vi "SRS SR124 Lockin.vi"(1 "Action":T5=enum."Identify", 2 "Parameters":variant) -> (6 "Output":variant, 7 "Stop":bool)   [LabVIEW 2025]
doc: "Author: Scott Hannahs <sth@magnet.fsu.edu>\n\nThis software is licensed for use under the “MIT License\"\nCopyright (c) 2025 Scott Hannahs, sth@sth@magnet.sthnet.net\n\nPermission is hereby granted, free of charge, to any person obtaining a copy of this software and associated documentation files (the \"Software\"), to deal in the Software without restriction, including without limitation the rights to use, copy, modify, merge, publish, distribute, sublicense, and/or sell copies of the Software, and to permit persons to whom the Software is furnished to do so, subject to the following conditions: The above copyright notice and this permission notice shall be included in all copies or substantial portions of the Software.\n\nTHE SOFTWARE IS PROVIDED \"AS IS\", WITHOUT WARRANTY OF ANY KIND, EXPRESS OR IMPLIED, INCLUDING BUT NOT LIMITED TO THE WARRANTIES OF MERCHANTABILITY, FITNESS FOR A PARTICULAR PURPOSE AND NONINFRINGEMENT. IN NO EVENT SHALL THE AUTHORS OR COPYRIGHT HOLDERS BE LIABLE FOR ANY CLAIM, DAMAGES OR OTHER LIABILITY, WHETHER IN AN ACTION OF CONTRACT, TORT OR OTHERWISE, ARISING FROM, OUT OF OR IN CONNECTION WITH THE SOFTWARE OR THE USE OR OTHER DEALINGS IN THE SOFTWARE."
uses:
  Sub Controls/Instrument Actions.ctl
  Sub Controls/Public.ctl
  Sub Controls/Instrument Match.ctl
  SubVIs/Lockin Channels.ctl
  Sub Controls/Factory Reset.ctl
  Sub Controls/Scan Output.ctl
  Sub Controls/Instrument IDN.ctl
  Sub Controls/User Event Command.ctl
panel:
  in  "Factory Reset":T1
  out "Channel Index":i32
  in  "Channels":T2={"X"=TRUE, "X&Y"=FALSE, "R"=FALSE, "R & ϴ"=FALSE}
  out "Model 2":string
  in  "Optical Port":enum32{"Port 1", "Port 2", "Port 3", "Port 4"}(radio)
  out "Title":string="Stanford Research Analog Lockin"
  in  "VISA resource name":refnum<visa-resource-name>
  in  "Instruments":T3[](array[typedef])=[{"Model"="SR124", "Manufacturer"="Stanford_Research_Systems", "Term Character"="", "Wait Time (mS)"=0, "Wait for SRQ"=FALSE, "Type"="Lockin"}, {"Model"="SR2124", "Manufacturer"="Stanford_Research_Systems", "Term Character"="", "Wait Time (mS)"=0, "Wait for SRQ"=FALSE, "Type"="Lockin"}]
  out "Model":string
  in  "Address":u16(ring)
  in  "Public":T4
  out "Measurement":dbl[](array[numeric]) format="%^.3e"
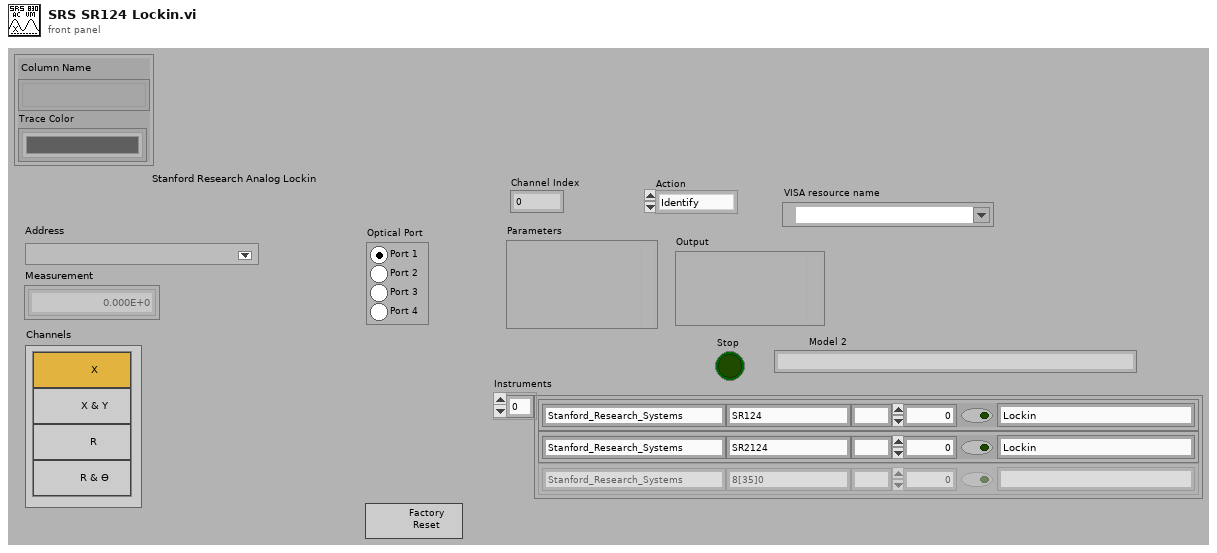
[diagram p1: front panel]
types:
  T1 = typedef "Factory Reset.ctl" = bool
  T2 = typedef "Lockin Channels.ctl" = cluster{"X":bool, "X&Y":bool, "R":bool, "R & ϴ":bool}
  T3 = typedef "Instrument Match.ctl" = cluster{"Model":string, "Manufacturer":string, "Term Character":string, "Wait Time (mS)":u32, "Wait for SRQ":bool, "Type":string}
  T4 = typedef "Public.ctl" = cluster{"Column Name":string[], "Trace Color":u32[]}
  T5 = typedef "Instrument Actions.ctl" = enum16{"Scan", "Identify", "New", "Configure", "Initialize", "Test", "Read", "Close"}
  T6 = typedef "Scan Output.ctl" = cluster{"Manufacturer":string, "Model":string, "Info":string, "Revision":string, "error out":errorcluster}
  T7 = typedef "Instrument IDN.ctl" = cluster{"VISA Address":string, "Status":u16, "Manufacturer":string, "Model":string, "Info":string, "Info 2":string, "Misc Data":variant}
  T8 = typedef "User Event Command.ctl" = enum32{"Stop Config"}
  T9 = typedef "Instrument Properties.ctl" = cluster{"Public":T4, "Private":T10}
  T10 = typedef "Private.ctl" = cluster{"Path":path, "VI Refnum":T11, "Name":string, "# of Values":i32, "Scale Factors":dbl[], "Display":T12[], "Offset":dbl[]}
  T11 = typedef "Instrument Ref.ctl" = refnum<vi>
  T12 = typedef "SystemCheckBox-resize.ctl" = bool
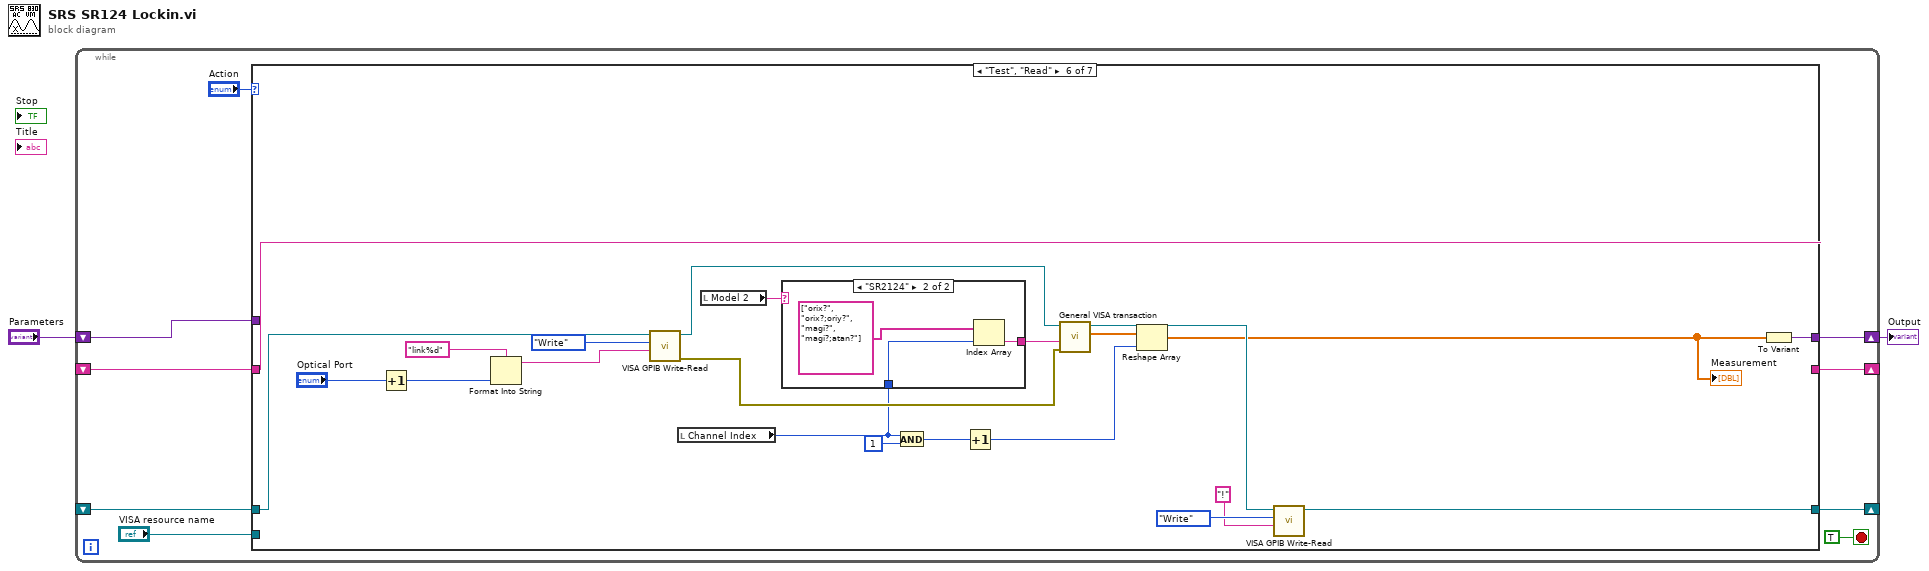
[diagram p0: block diagram]
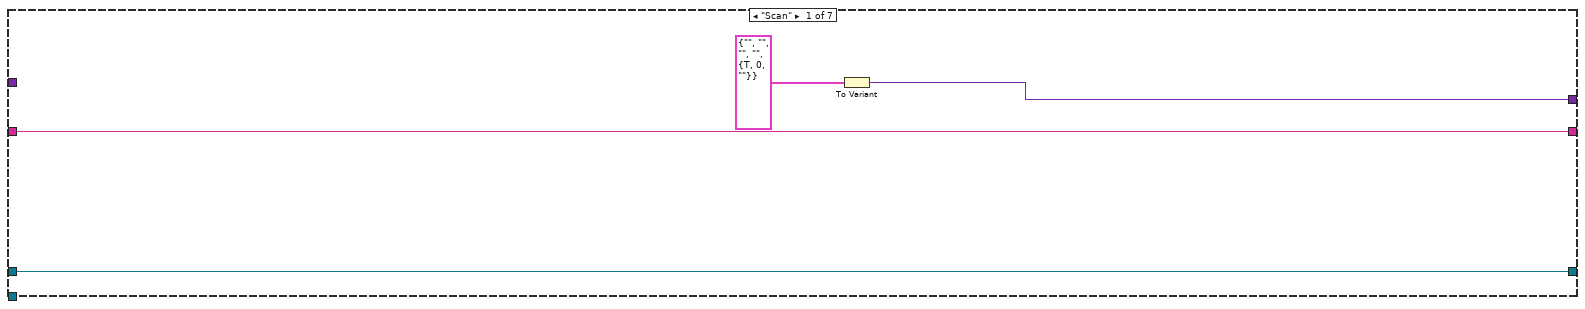
[diagram p2: hidden frame]
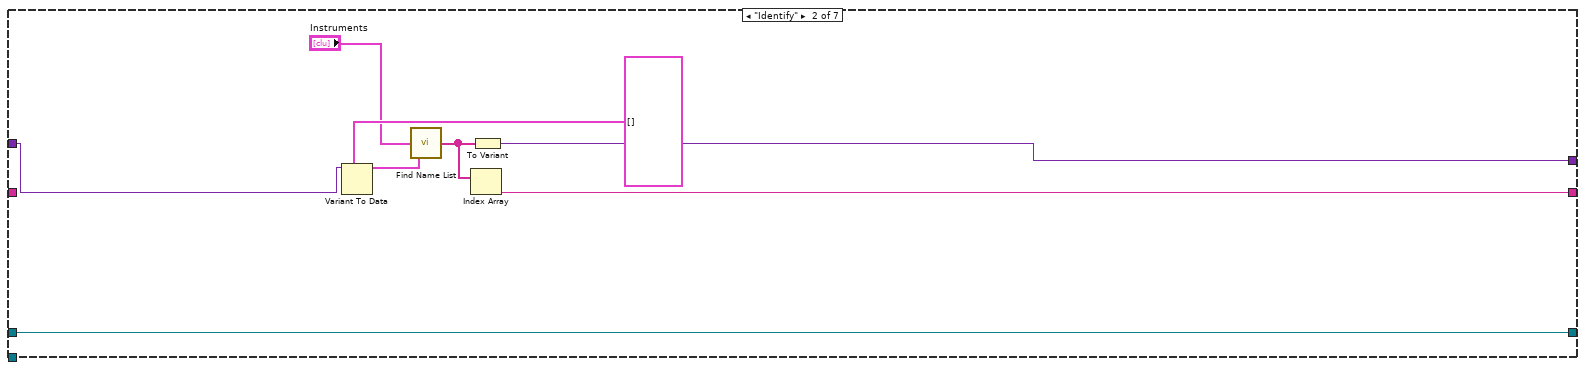
[diagram p3: hidden frame]
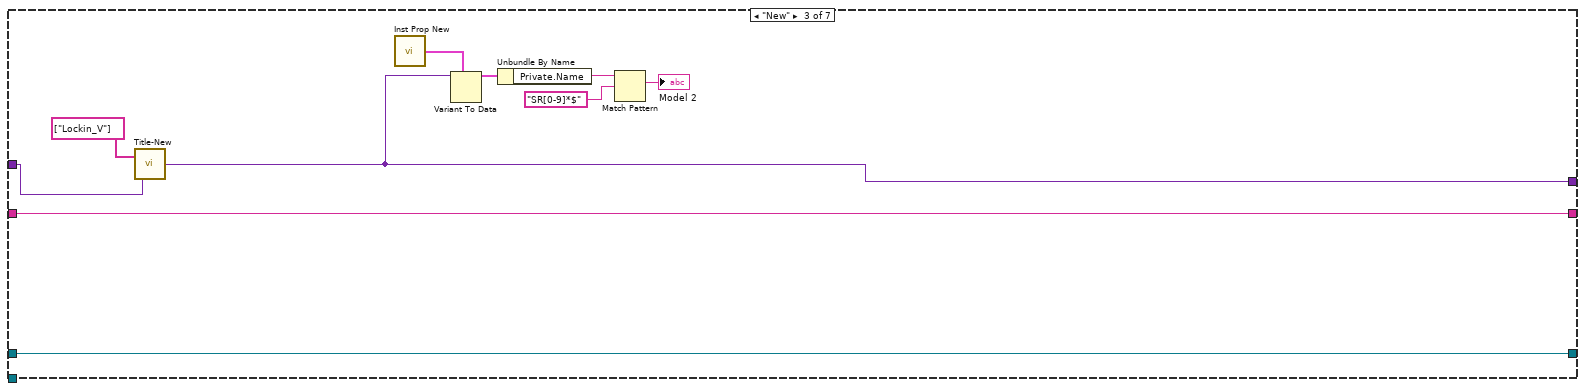
[diagram p4: hidden frame]
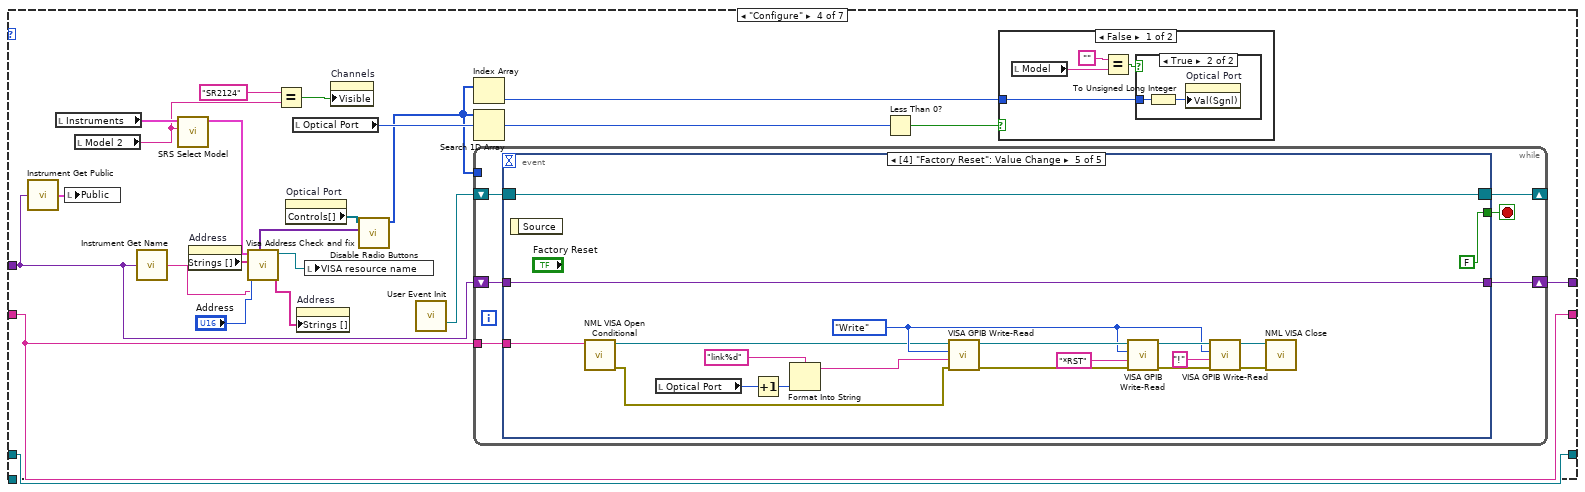
[diagram p5: hidden frame]
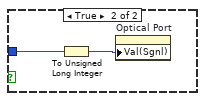
[diagram p7: hidden frame]
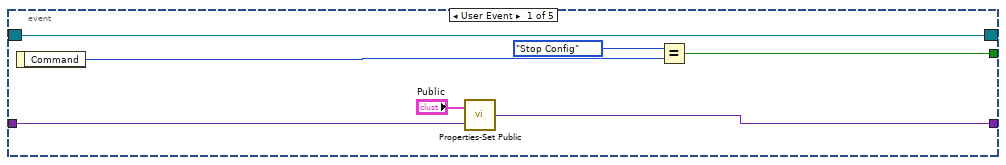
[diagram p8: hidden frame]
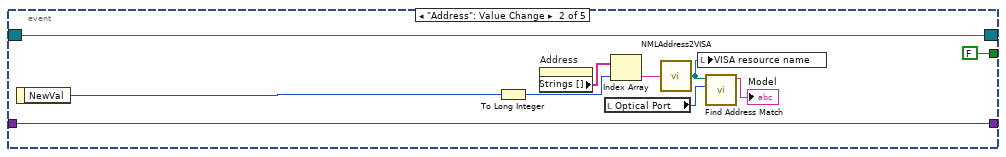
[diagram p9: hidden frame]
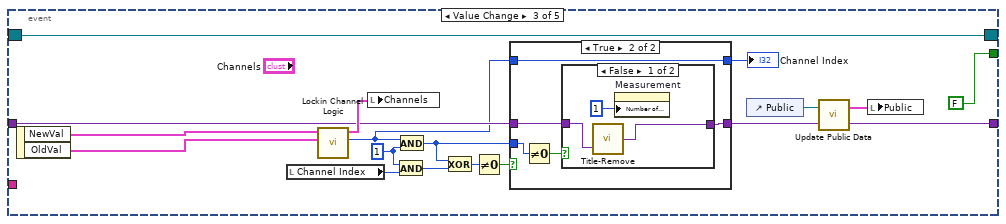
[diagram p10: hidden frame]
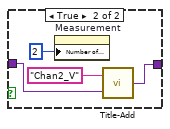
[diagram p12: hidden frame]
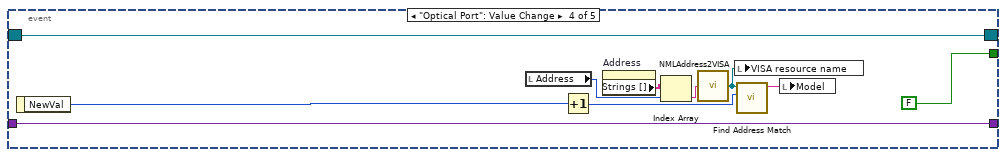
[diagram p13: hidden frame]
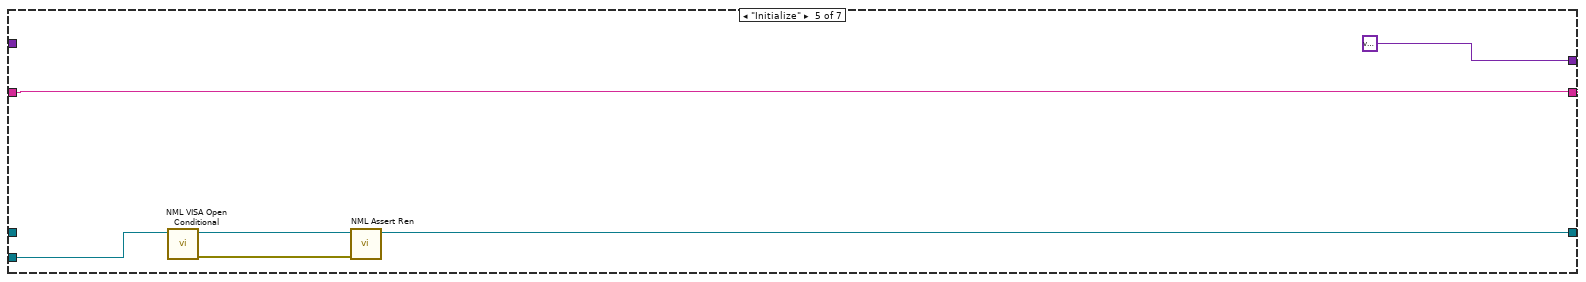
[diagram p14: hidden frame]
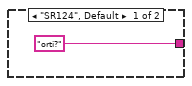
[diagram p15: hidden frame]
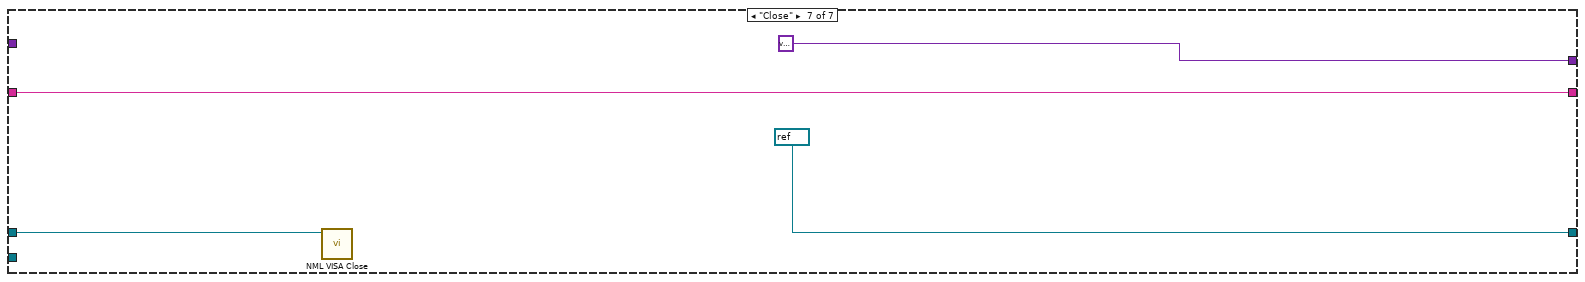
[diagram p16: hidden frame]
diagram:
  n1 = while {
    shift-right: [w10] -> _
    shift-left: _ -> [w9]
    shift-right: [w7] -> w1
    shift-left: "Parameters" -> [w8]
    shift-right: [w4] -> _
    shift-left: _ -> [w3]
    stop <- TRUE stop-if-true
    n2 = case shown="\"Test\", \"Read\"" "Action" {
      tunnel: [w14 w23 w32 w56 w150 w169 refnum<visa-resource-name> refnum ("Open VISA Resource name")] -> w10
      tunnel: w9 -> [w14 w23 w32 w56 _ w174 w181]
      tunnel: w8 -> [_ w20 w33 w47 _ _ _]
      tunnel: [w13 w22 w28 w55 variant ("Variant") w176 variant ("Variant")] -> w7
      tunnel: "VISA resource name" -> [_ _ _ _ w149 _ _]
      tunnel: [w12 w16 w30 w34 w153 w175 w182] -> w4
      tunnel: w3 -> [w12 _ w30 w34 w153 w175 w182]
      frame "Scan" {
        n3 = To Variant(anything=T6 {"Manufacturer"="", "Model"="", "Info"="", "Revision"="", "error out"={"status"=TRUE, "code"=0, "source"=""}} ("Scan Output")) -> (Variant=w13:variant)
      }
      frame "Identify" {
        n4 = Variant To Data(type=T7[] [], Variant=w20) -> (data=w18:T7[])  [unwired: 1 in, 1 out]
        n5 = call "Find Name List.vi"("Bus Scan"=w18, "Instruments"="Instruments") -> ("Names"=w17:string[])  [unwired: 1 in]
        n6 = Index Array(array=w17) -> (element=w16:string)  [unwired: 1 in]
        n7 = To Variant(anything=w17) -> (Variant=w22:variant)
      }
      frame "New" {
        n8 = call "Title-New.vi"("Parameters"=w33, "Array"=string[] ["Lockin_V"]) -> ("Instrument Prop"=w28:variant)
        n9 = call "Inst Prop New.vi"() -> ("Instrument Prop Out"=w29:T9)
        n10 = Variant To Data(type=w29, Variant=w28) -> (data=w27:T9)  [unwired: 1 in, 1 out]
        n11 = Unbundle By Name(w27) -> ("Private.Name"=w26:string)
        n12 = Match Pattern(string=w26, regular expression="SR[0-9]*$") -> (match substring=→"Model 2":string)  [unwired: 1 in, 3 out]
      }
      frame "Configure" {
        n13 = call "Instrument Get Public.vi"("Variant"=w47) -> ("Public"=w54:T4)
        n14 = local read "Instruments"() -> (w39:T3[])
        n15 = local write "Public"(w54) -> ()
        n16 = local read "Model 2"() -> (w35:string)
        n17 = call "Instrument Get Name.vi"("Parameters"=w47) -> ("Type"=w48:string)
        n18 = call "SRS Select Model.vi"("Model"=w35, "Instruments in"=w39) -> ("Instruments out"=w38:T3[])  [unwired: 9 in]
        n19 = property on="Address" class="Ring (strict)"() -> ("Strings []"=w51:string[])  [unwired: 2 in, 2 out]
        n20 = call "Visa Address Check and fix.vi"("Instruments"=w38, "NML Addresses"=w51, "Name"=w48, "Address"="Address") -> ("Array"=w46:variant[], "VISA resource name"=w50:refnum<visa-resource-name>, "NML Addresses"=w49:string[])  [unwired: 4 out]
        n21 = Equal?(x="SR2124", y=w35) -> (x = y?=w37:bool)
        n22 = property on="Optical Port" class="RadioBtnsControl (strict)"() -> ("Controls[]"=w45:refnum<vi>[])  [unwired: 2 in, 2 out]
        n23 = local read "Optical Port"() -> (w42:enum32{"Port 1", "Port 2", "Port 3", "Port 4"})
        n24 = property on="Address" class="Ring (strict)"("Strings []"=w49) -> ()  [unwired: 2 in, 2 out]
        n25 = local write "VISA resource name"(w50) -> ()
        n26 = property on="Channels" class="Clust (strict)"("Visible"=w37) -> ()  [unwired: 2 in, 2 out]
        n27 = call "Disable Radio Buttons.vi"("Array in"=w46, "Controls[]"=w45) -> ("Array out"=w41:i32[])  [unwired: 9 in]
        n28 = call "User Event Init.vi"() -> ("Event Registration Refnum"=w53:refnum<event-registration>)  [unwired: 14 in, 1 out]
        n29 = Index Array(array=w41) -> (element=w40:i32)  [unwired: 1 in]
        n30 = Search 1D Array(1D array=w41, element=w42) -> (index of element=w44:i32)  [unwired: 1 in]
        n31 = while {
          shift-right: [w70] -> w55
          shift-left: w47 -> [w69]
          shift-right: [w66] -> _
          shift-left: w53 -> [w67]
          tunnel: w41 -> [_]
          tunnel: w34 -> [w65]
          stop <- w68 stop-if-true
          n32 = event shown="[4] \"Factory Reset\": Value Change" {
            selector: w67 -> [w71 w87 w101 w129 w148]
            dyn-events: [w71 w87 w101 w129 w148] -> w66
            timeout: _ -> [_ _ _ _ _]
            tunnel: [w73 FALSE FALSE FALSE FALSE] -> w68
            tunnel: w69 -> [w76 w81 w93 w125 w147]
            tunnel: [w77 w81 w104 w125 w147] -> w70
            tunnel: w65 -> [_ _ _ _ w132]
            event User Event {
              n33 = event-data() -> ("Command"=w75:T8)  [unwired: 1 in]
              n34 = call "Properties-Set Public.vi"("Variant"=w76, "New Public"="Public") -> ("Variant 2"=w77:variant)
              n35 = Equal?(x=User_Event_Command."Stop Config", y=w75) -> (x = y?=w73:bool)
            }
            event "Address": Value Change {
              n36 = event-data() -> ("NewVal"=w85:u16)  [unwired: 1 in]
              n37 = To Long Integer(number=w85) -> (32bit integer=w79:i32)
              n38 = property on="Address" class="Ring (strict)"() -> ("Strings []"=w84:string[])  [unwired: 2 in, 2 out]
              n39 = local read "Optical Port"() -> (w78:enum32{"Port 1", "Port 2", "Port 3", "Port 4"})
              n40 = Index Array(array=w84, index=w79) -> (element=w83:string)
              n41 = call "NMLAddress2VISA.vi"("NML Address"=w83) -> ("VISA resource name"=w80:refnum<visa-resource-name>)
              n42 = local write "VISA resource name"(w80) -> ()
              n43 = call "Find Address Match.vi"("Misc Info"=w78, "VISA resource name"=w80) -> ("Model"=→"Model":string)  [unwired: 2 in, 3 out]
            }
            event Value Change {
              w98 = 1 ("y")
              n44 = event-data() -> ("NewVal"=w95:T2, "OldVal"=w94:T2)  [unwired: 1 in]
              n45 = local read "Channel Index"() -> (w99:i32)
              n46 = call "Lockin Channel Logic.vi"("Old Channels"=w94, "New Channels"=w95) -> ("index of element"=w90:i32, "Channels Out"=w100:T2)  [unwired: 8 in]
              n47 = local write "Channels"(w100) -> ()
              n48 = And(x=w98, y=w99) -> (x .and. y?=w97:i32)
              n49 = And(x=w90, y=w98) -> (x .and. y?=w91:i32)
              n50 = Exclusive Or(1:w97, 2:w91) -> (0:w96:i32)
              n51 = Not Equal To 0?(x=w96) -> (x != 0?=w92:bool)
              n52 = case shown="True" w92 {
                tunnel: w93 -> [w106 w112]
                tunnel: [w106 w111] -> w89
                tunnel: w91 -> [_ w109]
                tunnel: [w107 w108] -> w88
                tunnel: w90 -> [w107 w108]
                frame False {
                }
                frame True {
                  n53 = Not Equal To 0?(x=w109) -> (x != 0?=w110:bool)
                  n54 = case shown="False" w110 {
                    tunnel: w112 -> [w115 w119]
                    tunnel: [w114 w118] -> w111
                    frame False {
                      n55 = call "Title-Remove.vi"("Parameters"=w115) -> ("Variant"=w114:variant)  [unwired: 1 in]
                      n56 = property on="Measurement" class="Arr (strict)"("Number of Columns"=u32 1) -> ()  [unwired: 2 in, 2 out]
                    }
                    frame True {
                      n57 = property on="Measurement" class="Arr (strict)"("Number of Columns"=u32 2) -> ()  [unwired: 2 in, 2 out]
                      n58 = call "Title-Add.vi"("Parameters"=w119, "String"="Chan2_V") -> ("Variant"=w118:variant)
                    }
                  }
                }
              }
              "Channel Index" <- w88
              n59 = control-ref of="Public"() -> (w103:refnum<vi>)
              n60 = call "Update Public Data.vi"("Variant In"=w89, "Public 2"=w103) -> ("Variant Out"=w104:variant, "Public"=w102:T4)
              n61 = local write "Public"(w102) -> ()
            }
            event "Optical Port": Value Change {
              n62 = event-data() -> ("NewVal"=w122:enum32{"Port 1", "Port 2", "Port 3", "Port 4"})  [unwired: 1 in]
              n63 = local read "Address"() -> (w123:u16)
              n64 = Increment(x=w122) -> (x+1=w121:enum32{"Port 1", "Port 2", "Port 3", "Port 4"})
              n65 = property on="Address" class="Ring (strict)"() -> ("Strings []"=w127:string[])  [unwired: 2 in, 2 out]
              n66 = Index Array(array=w127, index=w123) -> (element=w126:string)
              n67 = call "NMLAddress2VISA.vi"("NML Address"=w126) -> ("VISA resource name"=w124:refnum<visa-resource-name>)
              n68 = local write "VISA resource name"(w124) -> ()
              n69 = call "Find Address Match.vi"("Misc Info"=w121, "VISA resource name"=w124) -> ("Model"=w120:string)  [unwired: 2 in, 3 out]
              n70 = local write "Model"(w120) -> ()
            }
            event Value Change {
              w136 = enum16{"Write", "Read", "Write & Read"}."Write" ("Action")
              n71 = event-data() -> ()  [unwired: 1 in, 1 out]
              n72 = call "NML VISA Open Conditional.vi"("VISA resource name"=w132) -> ("error out"=w130:errorcluster, "dup VISA Session"=w131:refnum<visa-resource-name>)  [unwired: 8 in, 1 out]
              n73 = local read "Optical Port"() -> (w141:enum32{"Port 1", "Port 2", "Port 3", "Port 4"})
              n74 = Increment(x=w141) -> (x+1=w142:enum32{"Port 1", "Port 2", "Port 3", "Port 4"})
              n75 = Format Into String(format string="link%d", w142) -> (resulting string=w143:string)  [unwired: 2 in, 1 out]
              n76 = call "VISA GPIB Write-Read.vi"("error in (no error)"=w130, "Command"=w143, "Action"=w136, "VISA resource name"=w131) -> ("error out"=w135:errorcluster, "dup VISA Session"=w140:refnum<visa-resource-name>)  [unwired: 4 in, 2 out]
              n77 = call "VISA GPIB Write-Read.vi"("error in (no error)"=w135, "Command"="*RST", "Action"=w136, "VISA resource name"=w140) -> ("error out"=w134:errorcluster, "dup VISA Session"=w137:refnum<visa-resource-name>)  [unwired: 4 in, 2 out]
              n78 = call "VISA GPIB Write-Read.vi"("error in (no error)"=w134, "Command"="!", "Action"=w136, "VISA resource name"=w137) -> ("error out"=w133:errorcluster, "dup VISA Session"=w138:refnum<visa-resource-name>)  [unwired: 4 in, 2 out]
              n79 = call "NML VISA Close.vi"("Error In"=w133, "VISA resource name"=w138) -> ()  [unwired: 9 in, 1 out]
            }
          }
        }
        n80 = Less Than 0?(x=w44) -> (x < 0?=w43:bool)
        n81 = case shown="False" w43 {
          tunnel: w40 -> [w57 w63]
          frame False {
            n82 = local read "Model"() -> (w60:string)
            n83 = Equal?(x="", y=w60) -> (x = y?=w58:bool)
            n84 = case shown="True" w58 {
              tunnel: w57 -> [_ w61]
              frame False {
              }
              frame True {
                n85 = To Unsigned Long Integer(number=w61) -> (unsigned 32bit integer=w62:u32)
                n86 = property on="Optical Port" class="RadioBtnsControl (strict)"("Val(Sgnl)"=w62) -> ()  [unwired: 2 in, 2 out]
              }
            }
          }
          frame True {
            n87 = To Unsigned Long Integer(number=w63) -> (unsigned 32bit integer=w64:u32)
            n88 = property on="Optical Port" class="RadioBtnsControl (strict)"("Val(Sgnl)"=w64) -> ()  [unwired: 2 in, 2 out]
          }
        }
      }
      frame "Initialize" {
        n89 = call "NML VISA Open Conditional.vi"("VISA resource name"=w149) -> ("error out"=w151:errorcluster, "dup VISA Session"=w152:refnum<visa-resource-name>)  [unwired: 8 in, 1 out]
        n90 = call "NML Assert Ren.vi"("error in (no error)"=w151, "VISA resource name"=w152) -> ("dup VISA Session"=w150:refnum<visa-resource-name>)  [unwired: 8 in, 1 out]
      }
      frame "Test", "Read" {
        n91 = Increment(x="Optical Port") -> (x+1=w166:enum32{"Port 1", "Port 2", "Port 3", "Port 4"})
        n92 = Format Into String(format string="link%d", w166) -> (resulting string=w171:string)  [unwired: 2 in, 1 out]
        n93 = call "VISA GPIB Write-Read.vi"("Command"=w171, "Action"=enum16{"Write", "Read", "Write & Read"}."Write", "VISA resource name"=w174) -> ("error out"=w162:errorcluster, "dup VISA Session"=w163:refnum<visa-resource-name>)  [unwired: 5 in, 2 out]
        n94 = local read "Channel Index"() -> (w160:i32)
        n95 = local read "Model 2"() -> (w165:string)
        n96 = case shown="\"SR2124\"" w165 {
          tunnel: ["orti?" ("t") w180] -> w161
          tunnel: w160 -> [_ w179]
          frame "SR124", Default {
          }
          frame "SR2124" {
            n97 = Index Array(array=string[] ["orix?", "orix?;oriy?", "magi?", "magi?;atan?"], index=w179) -> (element=w180:string)
          }
        }
        n98 = And(x=w160, y=1) -> (x .and. y?=w156:i32)
        n99 = Increment(x=w156) -> (x+1=w155:i32)
        n100 = call "General VISA transaction.vi"("error in (no error)"=w162, "Command String"=w161, "VISA Session"=w163) -> ("Measurement"=w158:dbl[], "dup VISA Session"=w164:refnum<visa-resource-name>)  [unwired: 3 in, 4 out]
        n101 = Reshape Array(w158, w155) -> (w157:dbl[])
        "Measurement" <- w157
        n102 = call "VISA GPIB Write-Read.vi"("Command"="!", "Action"=enum16{"Write", "Read", "Write & Read"}."Write", "VISA resource name"=w164) -> ("dup VISA Session"=w169:refnum<visa-resource-name>)  [unwired: 5 in, 3 out]
        n103 = To Variant(anything=w157) -> (Variant=w176:variant)
      }
      frame "Close" {
        n104 = call "NML VISA Close.vi"("VISA resource name"=w181) -> ()  [unwired: 10 in, 1 out]
      }
    }
  }
  "Output" <- w1
